vi "Create New Handler.vi"(7 "Handler type":refnum<class "Handler.lvclass">, 8 "error in (no error)":errorcluster, 10 "Name":string, 11 "Level":T1(ring)) -> (0 "error out":errorcluster, 3 "Handler":refnum<class "Handler.lvclass">)   [LabVIEW 2017, in "Error Log.lvlib" / "Handler.lvclass"]
doc: "Creates a new <b>Handler</b> nammed <b>Name</b> to log message with severity equal or higher than <b>Level</b>."
uses:
  Handler.lvclass
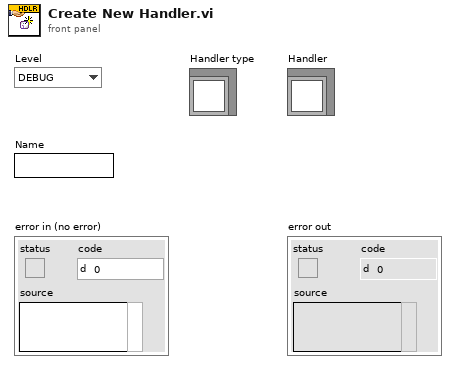
[diagram p1: front panel]
types:
  T1 = enum16{"DEBUG", "INFO", "WARNING", "ERROR", "CRITICAL"}
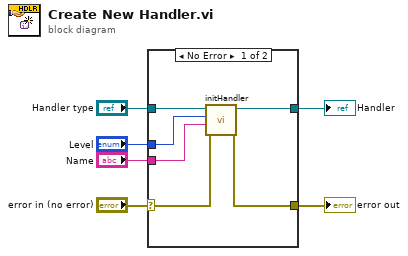
[diagram p0: block diagram]
diagram:
  n1 = case shown="No Error" "error in (no error)" {
    selector: "error in (no error)" -> [w10 w14]
    tunnel: [w9 w14] -> w5
    tunnel: [w11 w13] -> w3
    tunnel: "Handler type" -> [w12 w13]
    tunnel: "Level" -> [w8 _]
    tunnel: "Name" -> [w7 _]
    frame No Error {
      n2 = call-dynamic "initHandler.vi"("error in (no error)"=w10, "Name"=w7, "Level"=w8, "Handler in"=w12) -> ("error out"=w9:errorcluster, "Handler out"=w11:refnum<class "Handler.lvclass">)  [unwired: 6 in]
    }
    frame Error {
    }
  }
  "error out" <- w5
  "Handler" <- w3
